vi "PrepareIESource.vi"() -> ()   [LabVIEW 2021]
uses:
  <vilib>/Wiresmith Technology/G CLI/CLI Class/CLI.lvclass
  <userlib>/_OpenG.lib/lvzip/lvzip.llb/subVI/ZLIB Compress Directory (Path)__ogtk.vi
  <userlib>/_OpenG.lib/lvzip/lvzip.llb/ZLIB Open ZIP Mode__ogtk.ctl
  <userlib>/_OpenG.lib/file/file.llb/openg_file.lvlib
  <userlib>/_OpenG.lib/file/file.llb/Convert File Extension (Path)__ogtk.vi
  <userlib>/_OpenG.lib/lvzip/fileutil.llb/subVIs/FILE Rename (Path)__ogtk.vi
panel:
  out "error out":errorcluster
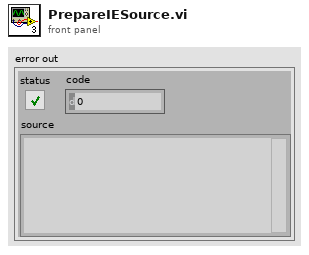
[diagram p1: front panel]
types:
  T1 = typedef "ZLIB Open ZIP Mode__ogtk.ctl" = enum16{"create new", "append to end", "append to archive"}
  T2 = enum32{"Invalid", "Standard", "Closed", "Hidden", "Minimized", "Maximized"}
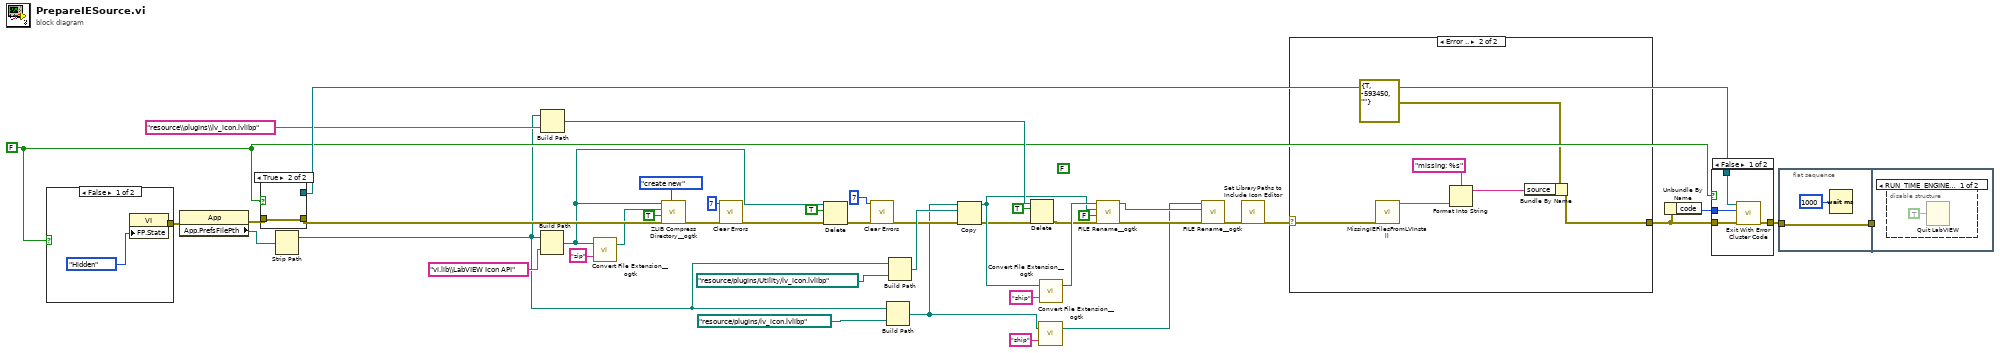
[diagram p0: block diagram]
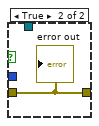
[diagram p3: hidden frame]
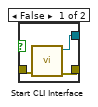
[diagram p5: hidden frame]
diagram:
  (unwired) FALSE ("cancelled")
  w20 = FALSE
  n1 = case shown="False" w20 {
    tunnel: [w44 _] -> w39
    frame False {
      n2 = property class="VI"("FP.State"=T2."Hidden" ("Front Panel Window:State")) -> (error out=w44:errorcluster)  [unwired: 2 in, 1 out]
    }
    frame True {
    }
  }
  n3 = property class="App"(error in=w39) -> (error out=w38:errorcluster, "App.PrefsFilePth"=w37:path)  [unwired: 1 in, 1 out]
  n4 = case shown="True" w20 {
    tunnel: [w48 _] -> w43
    tunnel: w38 -> [w47 w49]
    tunnel: [w46 w49] -> w32
    frame False {
      n5 = call <vilib>:"Start CLI Interface.vi"("error in (no error)"=w47) -> ("error out"=w46:errorcluster, "CLI out"=w48:refnum<class "CLI.lvclass">)  [unwired: 7 in, 2 out]
    }
    frame True {
    }
  }
  n6 = Strip Path(path=w37) -> (stripped path=w16:path)  [unwired: 1 out]
  n7 = Build Path(base path=w16, name or relative path="vi.lib\\LabVIEW Icon API" ("name")) -> (appended path=w27:path)
  n8 = Build Path(base path=w16, name or relative path="resource\\plugins\\lv_icon.lvlibp" ("name")) -> (appended path=w26:path)
  n9 = call-poly <userlib>:"Convert File Extension__ogtk.vi"("new ending (none)"="zip", "file name"=w27) -> ("new filename"=w30:path)  [unwired: 1 out]
  n10 = call-poly <userlib>:"ZLIB Compress Directory__ogtk.vi"("append (create new)"=ZLIB_Open_ZIP_Mode__ogtk."create new", "error in (no error)"=w32, "include subdirectories (F)"=TRUE, "archive name (root directory with .zip ending)"=w30, "root directory (file dialog)"=w27) -> ("error out"=w29:errorcluster)  [unwired: 4 in, 2 out]
  n11 = call <vilib>:"Clear Errors.vi"("error in (no error)"=w29, "specific error code to clear (0: all)"=7) -> ("error out"=w25:errorcluster)  [unwired: 4 in, 1 out]
  n12 = Delete(path (use dialog)=w27, entire hierarchy (F)=TRUE, error in=w25) -> (error out=w21:errorcluster)  [unwired: 2 in, 2 out]
  n13 = call <vilib>:"Clear Errors.vi"("error in (no error)"=w21, "specific error code to clear (0: all)"=7) -> ("error out"=w11:errorcluster)  [unwired: 4 in, 1 out]
  n14 = Build Path(base path=w16, name or relative path=path "resource/plugins/lv_icon.lvlibp") -> (appended path=w4:path)
  n15 = Build Path(base path=w16, name or relative path=path "resource/plugins/Utility/lv_icon.lvlibp") -> (appended path=w14:path)
  n16 = Copy(8:w11, 10:w14, 11:w4) -> (0:w10:errorcluster, 3:w12:path)  [unwired: 2 in, 1 out]
  n17 = Delete(path (use dialog)=w26, entire hierarchy (F)=TRUE, error in=w10) -> (error out=w9:errorcluster)  [unwired: 2 in, 2 out]
  n18 = call-poly <userlib>:"Convert File Extension__ogtk.vi"("new ending (none)"="ship", "file name"=w4) -> ("new filename"=w3:path)  [unwired: 1 out]
  n19 = call-poly <userlib>:"Convert File Extension__ogtk.vi"("new ending (none)"="ship", "file name"=w12) -> ("new filename"=w13:path)  [unwired: 1 out]
  n20 = call-poly <userlib>:"FILE Rename__ogtk.vi"("error in (no error)"=w9, "overwrite (F)"=FALSE, "source path"=w12, "target path"=w13) -> ("error out"=w8:errorcluster, "dup target path"=w6:path)  [unwired: 6 in]
  n21 = call-poly <userlib>:"FILE Rename__ogtk.vi"("error in (no error)"=w8, "source path"=w6, "target path"=w3) -> ("error out"=w7:errorcluster)  [unwired: 7 in, 1 out]
  n22 = call "Set LibraryPaths to Include Icon Editor.vi"("error in (no error)"=w7) -> ("error out"=w1:errorcluster)  [unwired: 9 in, 1 out]
  n23 = case shown="Error .." w1 {
    selector: w1 -> [w50 w56]
    tunnel: [w50 w53] -> w2
    frame No Error {
    }
    frame Error {
      n24 = call "MissingIEFilesFromLVInstall.vi"("error in (no error)"=w56) -> ("Missing IE Paths"=w51:string)  [unwired: 8 in, 2 out]
      n25 = Format Into String(format string="missing: %s", w51) -> (resulting string=w54:string)  [unwired: 2 in, 1 out]
      n26 = Bundle By Name(cluster=errorcluster {"status"=TRUE, "code"=-593450, "source"=""} ("error out"), "source"=w54) -> (w53:errorcluster)
    }
  }
  n27 = Unbundle By Name(w2) -> ("code"=w40:i32)
  n28 = case shown="False" w20 {
    tunnel: w43 -> [w60 _]
    tunnel: [w59 w61] -> w41
    tunnel: w40 -> [w58 _]
    tunnel: w2 -> [w57 w61]
    frame False {
      n29 = call <vilib>:"Exit With Error Cluster Code.vi"("error in (no error)"=w57, "No Error Code (0)"=w58, "CLI in"=w60) -> ("error out"=w59:errorcluster)  [unwired: 8 in]
    }
    frame True {
      "error out" <- w61
    }
  }
  n30 = flat-sequence {
    tunnel: w41 -> [w63]
    tunnel: [w63] -> w42
    tunnel: w42 -> [_]
    frame #0 {
      n31 = Wait (ms)(milliseconds to wait=u32 1000) -> ()  [unwired: 1 out]
    }
    frame #1 {
      n32 = disable-structure shown="RUN_TIME_ENGINE==True" {
        frame condition #0 {
          n33 = Quit LabVIEW(quit? (T)=TRUE) -> ()
        }
        frame condition #1 (active) {
        }
      }
    }
  }
